vi "Serial_Write_Read_xbox_Polling.vi"() -> ()   [LabVIEW 2023]
uses:
  <vilib>/MakerHub/Xbox-One-Controller/Private/Type Defs/Indicators/Controller.ctl
  <vilib>/MakerHub/Xbox-One-Controller/Private/Type Defs/Indicators/A.ctl
  <vilib>/MakerHub/Xbox-One-Controller/Private/Type Defs/Indicators/B.ctl
  <vilib>/MakerHub/Xbox-One-Controller/Private/Type Defs/Indicators/X.ctl
  <vilib>/MakerHub/Xbox-One-Controller/Private/Type Defs/Indicators/Y.ctl
  <vilib>/MakerHub/Xbox-One-Controller/Private/Type Defs/Indicators/Left Bumper.ctl
  <vilib>/MakerHub/Xbox-One-Controller/Private/Type Defs/Indicators/Right Bumper.ctl
  <vilib>/MakerHub/Xbox-One-Controller/Private/Type Defs/Indicators/View.ctl
  <vilib>/MakerHub/Xbox-One-Controller/Private/Type Defs/Indicators/Menu.ctl
  <vilib>/MakerHub/Xbox-One-Controller/Private/Type Defs/Indicators/Thumbstick_Analog.ctl
  <vilib>/MakerHub/Xbox-One-Controller/Private/Type Defs/Indicators/Slider.ctl
  <vilib>/MakerHub/Xbox-One-Controller/Private/Type Defs/Indicators/DPad.ctl
  <vilib>/MakerHub/Xbox-One-Controller/Public/Open First Controller.vi
  <vilib>/Instr/_visa.llb/VISA Configure Serial Port (Instr).vi
  <vilib>/MakerHub/Xbox-One-Controller/LMH-Xbox-One-Controller.lvlib
panel:
  in  "Left Stick":u32(slide)=50 scale=0.0..100.0
  out "Loop Timer":i32
  out "Panel Outputs\nActive":bool
  in  "Right Bumper":T1 caption="Blank Button"
  in  "Left Bumper":T2 caption="Blank Button"
  in  "Menu Button":T3 caption="Blank Button"
  in  "View Button":T4 caption="Blank Button"
  in  "Y":T5 caption="Blank Button"
  in  "X":T6 caption="Blank Button"
  in  "B":T7 caption="Blank Button"
  in  "A":T8 caption="Blank Button"
  in  "Right Stick":u32(slide)=50 scale=0.1..100.0
  in  "Panel Buttons / Xbox Buttons":bool
  out "Controller":T9={"A Button"=FALSE, "B Button"=FALSE, "X Button"=FALSE, "Y Button"=FALSE, "Left Bumper"=FALSE, "Right Bumper"=FALSE, "View Button"=FALSE, "Menu Button"=FALSE, "Left Stick"={[], []}, "Right Stick"={[], []}, "Trigger"=0, "D-Pad"=5} {"Trigger" scale=32767.0..-32768.0}
  out "X Axis Right":u32
  out "X Axis Left":u32
  out "error out":errorcluster
  in  "error in (no error)":errorcluster
  in  "byte count\nRead":u32=40
  in  "Loop Timer":u32=100 min=10
  out "Concatenated \nNumber":string
  in  "VISA resource name":refnum<visa-resource-name>="COM3"
  out "byte count Sent":u32
  out "read buffer":string
  out "Controller Outputs\nActive":bool
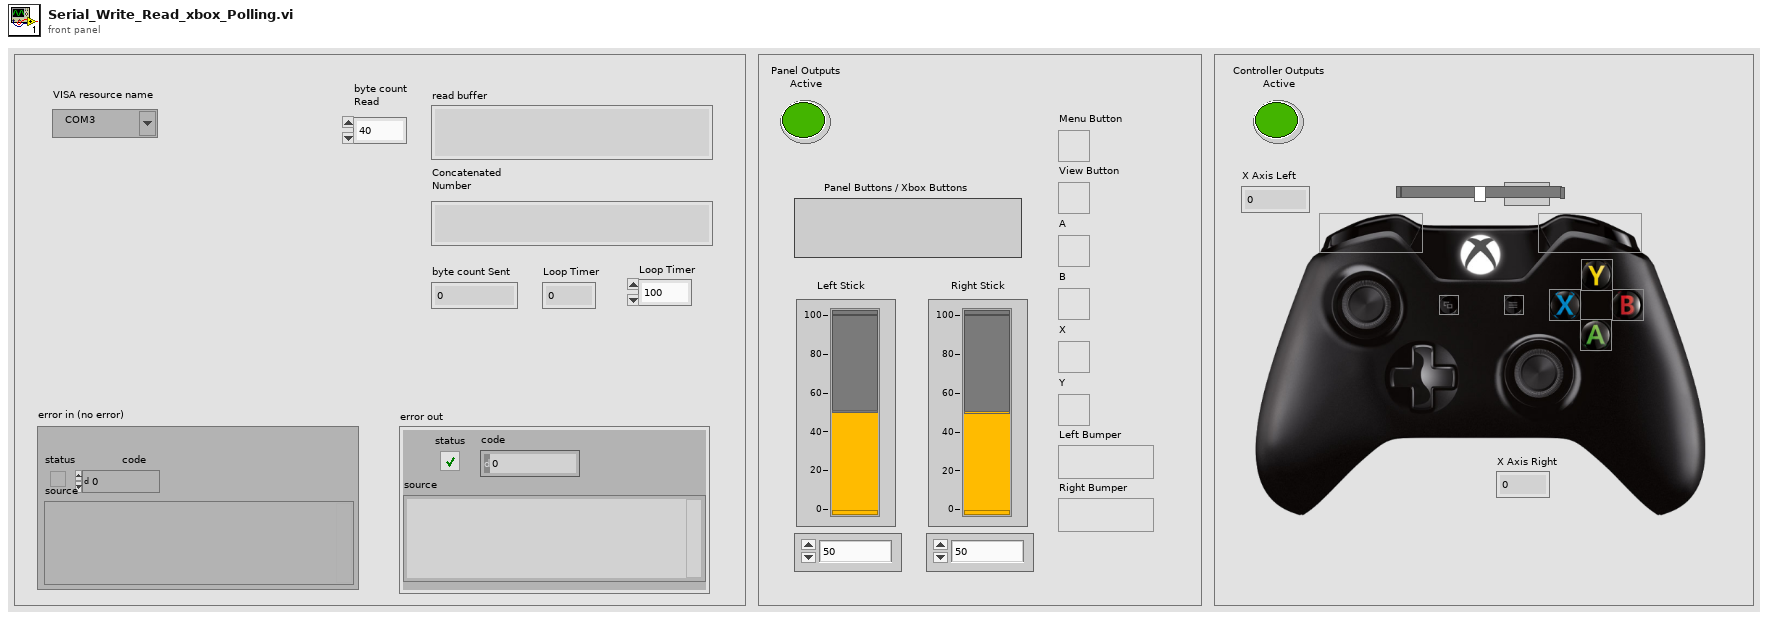
[diagram p1: front panel]
types:
  T1 = typedef "LMH-Xbox-One-Controller.lvlib/Right Bumper.ctl" = bool
  T2 = typedef "LMH-Xbox-One-Controller.lvlib/Left Bumper.ctl" = bool
  T3 = typedef "LMH-Xbox-One-Controller.lvlib/Menu.ctl" = bool
  T4 = typedef "LMH-Xbox-One-Controller.lvlib/View.ctl" = bool
  T5 = typedef "LMH-Xbox-One-Controller.lvlib/Y.ctl" = bool
  T6 = typedef "LMH-Xbox-One-Controller.lvlib/X.ctl" = bool
  T7 = typedef "LMH-Xbox-One-Controller.lvlib/B.ctl" = bool
  T8 = typedef "LMH-Xbox-One-Controller.lvlib/A.ctl" = bool
  T9 = typedef "LMH-Xbox-One-Controller.lvlib/Controller.ctl" = cluster{"A Button":T8, "B Button":T7, "X Button":T6, "Y Button":T5, "Left Bumper":T2, "Right Bumper":T1, "View Button":T4, "Menu Button":T3, "Left Stick":T10, "Right Stick":T10, "Trigger":T11, "D-Pad":T12}
  T10 = typedef "LMH-Xbox-One-Controller.lvlib/Thumbstick_Analog.ctl" = cluster{i32[], i32[]}
  T11 = typedef "LMH-Xbox-One-Controller.lvlib/Slider.ctl" = i32
  T12 = typedef "LMH-Xbox-One-Controller.lvlib/DPad.ctl" = u16
  T13 = typedef "LMH-Xbox-One-Controller.lvlib/Xbox One Controller Ref.ctl" = cluster{"Controller Ref":refnum<k1>, "Event Refnum":refnum<event-registration>, "Worker Ref":refnum<vi>}
  T14 = typedef "LMH-Xbox-One-Controller.lvlib/All Axis Data.ctl" = cluster{"Left Stick":cluster{"X Axis":i32, "Y Axis":i32}, "Right Stick":cluster{"X Axis":i32, "Y Axis":i32}, "Triggers":i32, "D-Pad":T15}
  T15 = typedef "LMH-Xbox-One-Controller.lvlib/DPad Enum.ctl" = enum16{"Idle", "Up", "Up / Right", "Right", "Down / Right", "Down", "Down / Left", "Left", "Up / Left"}
  T16 = typedef "LMH-Xbox-One-Controller.lvlib/All Buttons Visual.ctl" = cluster{"A":T8, "B":T7, "X":T6, "Y":T5, "Left Bumper":T2, "Right Bumper":T1, "View Button":T4, "Menu Button":T3, "Left Stick":T17, "Right Stick":T17}
  T17 = typedef "LMH-Xbox-One-Controller.lvlib/Thumbstick.ctl" = bool
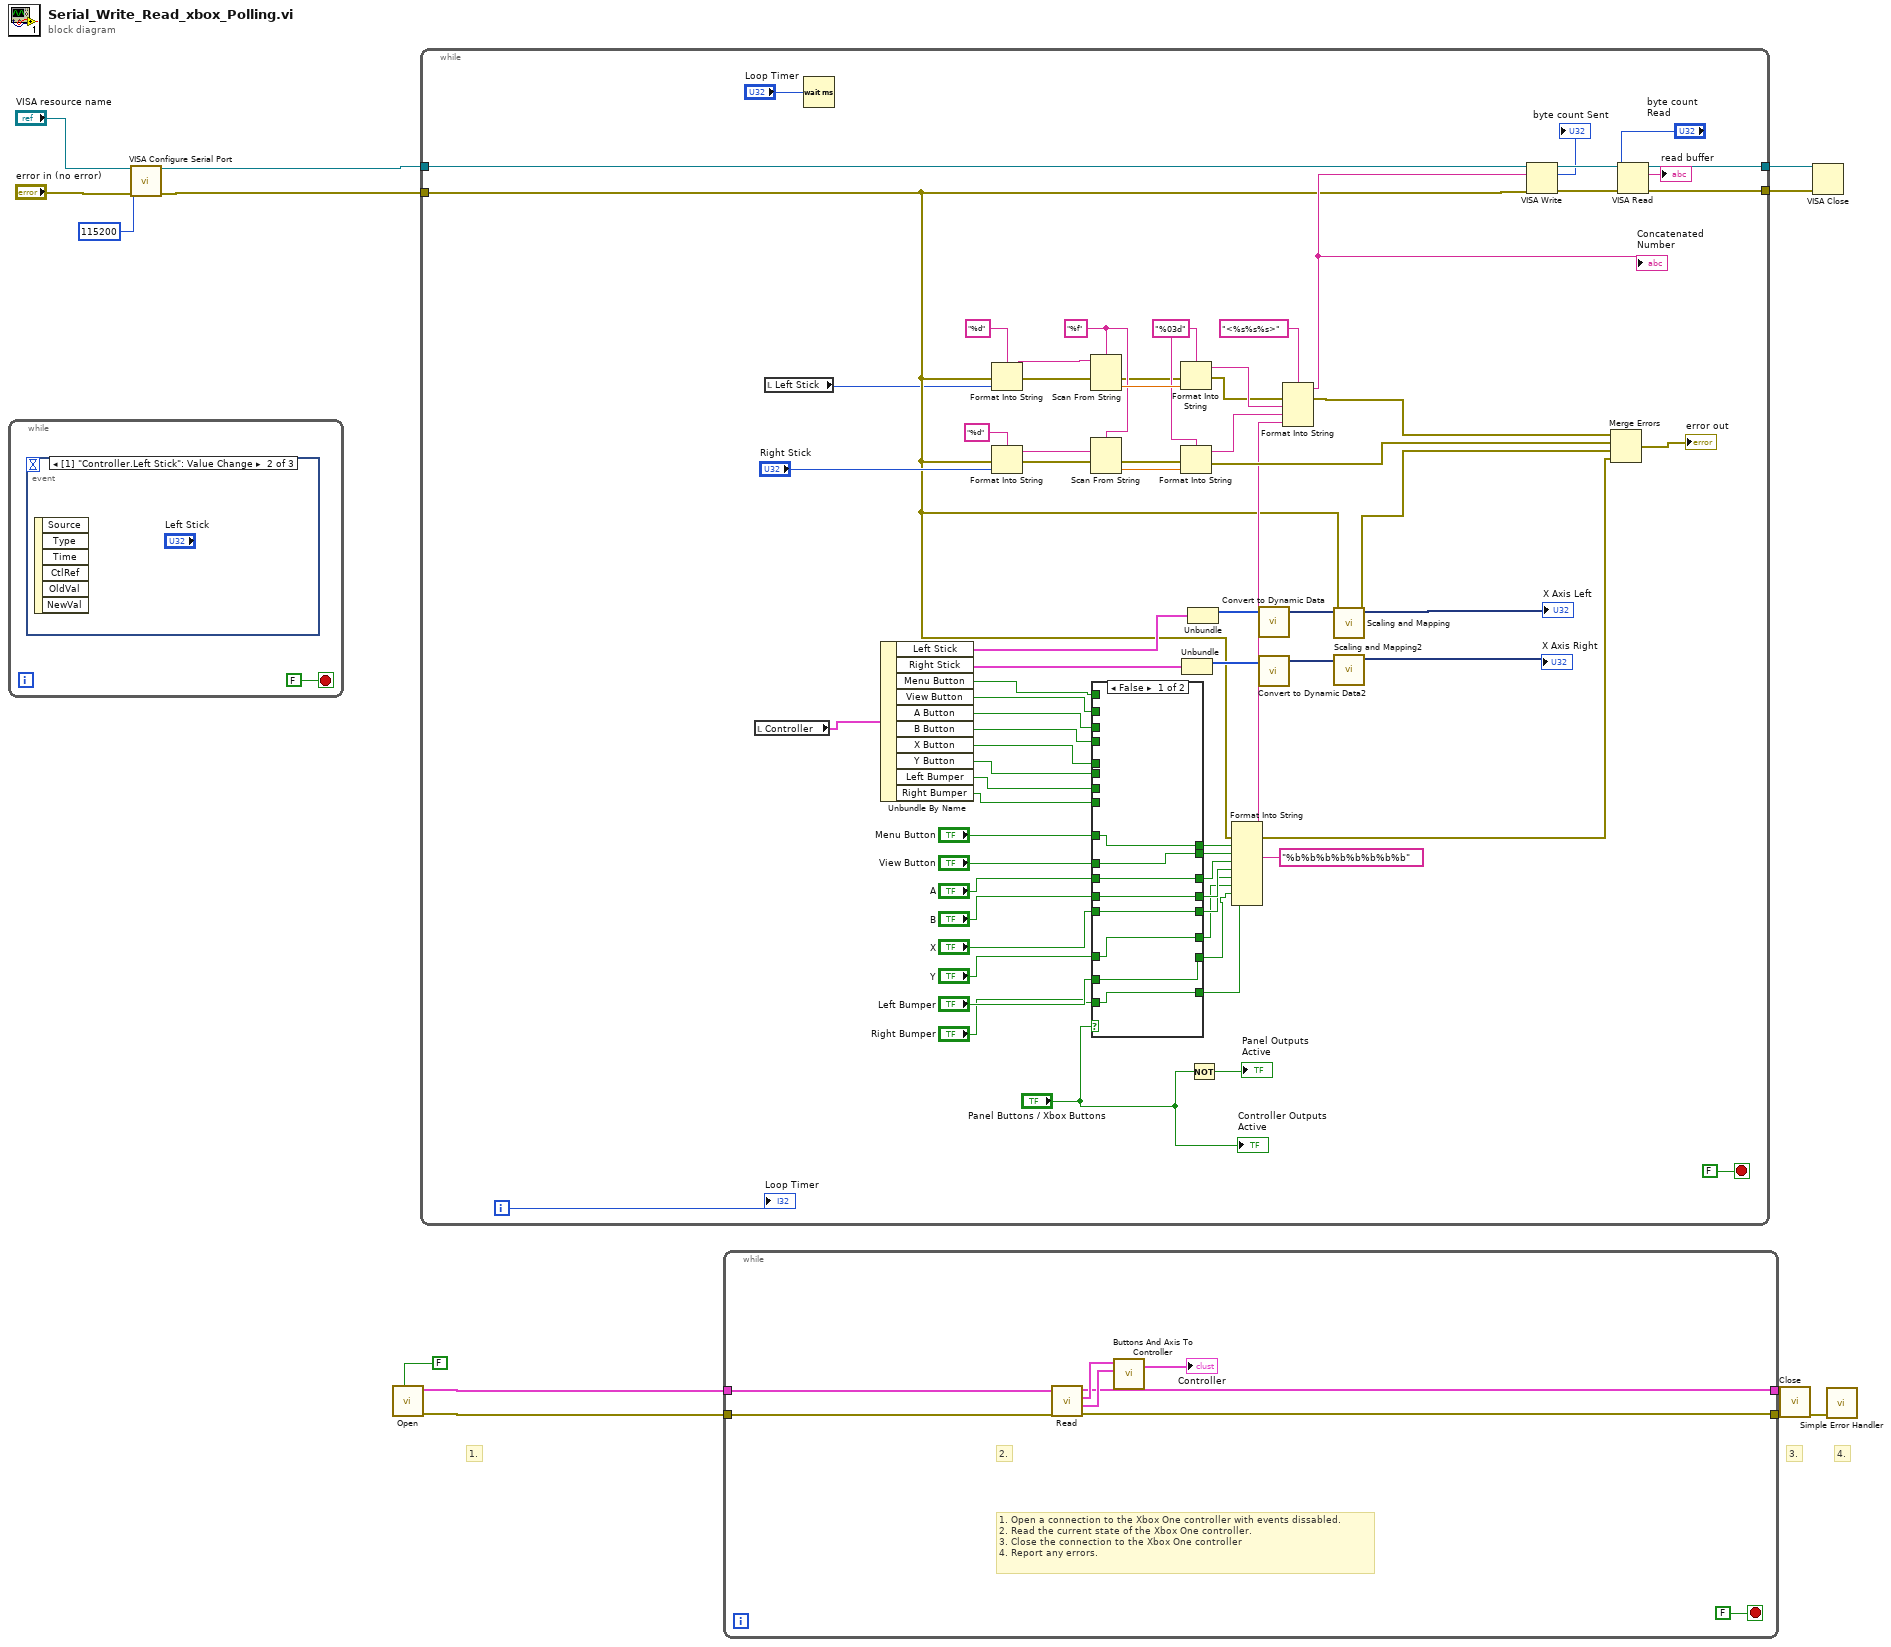
[diagram p0: block diagram]
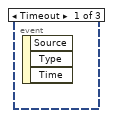
[diagram p2: hidden frame]
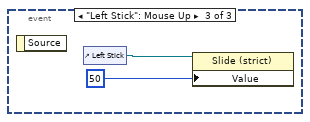
[diagram p3: hidden frame]
diagram:
  # "4."
  # "3."
  # "1."
  n1 = while {
    stop <- FALSE stop-if-true
    n2 = event shown="[1] \"Controller.Left Stick\": Value Change" {
      selector: _ -> [_ _ _]
      dyn-events: _ -> [_ _ _]
      timeout: _ -> [_ _ _]
      event Timeout {
        n3 = event-data() -> ()  [unwired: 1 in, 3 out]
      }
      event Value Change {
        n4 = event-data() -> ()  [unwired: 1 in, 6 out]
      }
      event "Left Stick": Mouse Up {
        n5 = event-data() -> ()  [unwired: 1 in, 1 out]
        n6 = control-ref of="Left Stick"() -> (w16:refnum<vi>)
        n7 = property class="Slide (strict)"(reference=w16, "Value"=u32 50) -> ()  [unwired: 1 in, 2 out]
      }
    }
  }
  n8 = call-poly "VISA Configure Serial Port"("VISA resource name"="VISA resource name", "baud rate (9600)"=u32 115200, "error in (no error)"="error in (no error)") -> ("VISA resource name out"=w11:refnum<visa-resource-name>, "error out"=w10:errorcluster)  [unwired: 11 in]
  n9 = call-poly <vilib>:"Open.vi"("Enable Events (T)"=FALSE) -> ("Error Out"=w4:errorcluster, "Xbox One Controller"=w3:T13)  [unwired: 8 in, 1 out]
  n10 = while {
    tunnel: [w88] -> w13
    tunnel: [w86] -> w12
    tunnel: w11 -> [w83]
    tunnel: w10 -> [w24]
    i -> [w22]
    stop <- FALSE stop-if-true
    w73 = "%f" ("format string")
    w75 = "%03d" ("format string")
    n11 = local read "Controller"() -> (w21:T9)
    n12 = local read "Left Stick"() -> (w17:u32)
    n13 = Wait (ms)(milliseconds to wait="Loop Timer") -> ()  [unwired: 1 out]
    n14 = Unbundle By Name(w21) -> ("Left Stick"=w60:T10, "Right Stick"=w59:T10, "Menu Button"=w33:T3, "View Button"=w32:T4, "A Button"=w31:T8, "B Button"=w30:T7, "X Button"=w29:T6, "Y Button"=w28:T5, "Left Bumper"=w27:T2, "Right Bumper"=w26:T1)
    n15 = Format Into String(format string="%d", error in=w24, w17) -> (resulting string=w79:string, error out=w68:errorcluster)  [unwired: 1 in]
    n16 = Format Into String(format string="%d", error in=w24, "Right Stick") -> (resulting string=w74:string, error out=w65:errorcluster)  [unwired: 1 in]
    n17 = Scan From String(format string=w73, input string=w79, error in=w68) -> (error out=w67:errorcluster, output 1=w80:dbl)  [unwired: 2 in, 2 out]
    n18 = Scan From String(format string=w73, input string=w74, error in=w65) -> (error out=w64:errorcluster, output 1=w70:dbl)  [unwired: 2 in, 2 out]
    n19 = case shown="False" "Panel Buttons / Xbox Buttons" {
      tunnel: "Menu Button" -> [w97 _]
      tunnel: [w97 w105] -> w48
      tunnel: "View Button" -> [w96 _]
      tunnel: [w96 w104] -> w46
      tunnel: "A" -> [w95 _]
      tunnel: [w95 w103] -> w44
      tunnel: "B" -> [w94 _]
      tunnel: "X" -> [w93 _]
      tunnel: "Y" -> [w92 _]
      tunnel: "Left Bumper" -> [w91 _]
      tunnel: "Right Bumper" -> [w90 _]
      tunnel: [w94 w102] -> w38
      tunnel: [w93 w101] -> w37
      tunnel: [w92 w100] -> w36
      tunnel: [w91 w99] -> w35
      tunnel: [w90 w98] -> w34
      tunnel: w33 -> [_ w105]
      tunnel: w32 -> [_ w104]
      tunnel: w31 -> [_ w103]
      tunnel: w30 -> [_ w102]
      tunnel: w29 -> [_ w101]
      tunnel: w28 -> [_ w100]
      tunnel: w27 -> [_ w99]
      tunnel: w26 -> [_ w98]
      frame False {
      }
      frame True {
      }
    }
    n20 = Format Into String(format string=w75, error in=w67, w80) -> (resulting string=w78:string, error out=w66:errorcluster)  [unwired: 1 in]
    n21 = Format Into String(format string=w75, error in=w64, w70) -> (resulting string=w76:string, error out=w62:errorcluster)  [unwired: 1 in]
    n22 = Unbundle(w59) -> (w54:i32[])  [unwired: 1 out]
    n23 = Unbundle(w60) -> (w58:i32[])  [unwired: 1 out]
    n24 = Not(x="Panel Buttons / Xbox Buttons") -> (.not. x?=→"Panel Outputs\nActive":bool)
    n25 = Format Into String(format string="%b%b%b%b%b%b%b%b", error in=w24, w48, w46, w44, w38, w37, w36, w35, w34) -> (resulting string=w51:string, error out=w23:errorcluster)  [unwired: 1 in]
    n26 = call "Convert to Dynamic Data"("Array"=w58) -> ("Dynamic Data Type"=w55:dynamicdata)  [unwired: 3 in]
    n27 = call "Convert to Dynamic Data2"("Array"=w54) -> ("Dynamic Data Type"=w53:dynamicdata)  [unwired: 3 in]
    n28 = Format Into String(format string="<%s%s%s>", error in=w66, w78, w76, w51) -> (resulting string=w69:string, error out=w63:errorcluster)  [unwired: 1 in]
    "Concatenated \nNumber" <- w69
    n29 = call "Scaling and Mapping"("error in (no error)"=w24, "Signals"=w55) -> ("error out"=w56:errorcluster, "Scaled Signals"=→"X Axis Left":dynamicdata)  [unwired: 8 in]
    n30 = call "Scaling and Mapping2"("Signals"=w53) -> ("Scaled Signals"=→"X Axis Right":dynamicdata)  [unwired: 9 in, 1 out]
    n31 = VISA Write(VISA resource name=w83, write buffer=w69, error in (no error)=w24) -> (VISA resource name out=w89:refnum<visa-resource-name>, return count=→"byte count Sent":u32, error out=w85:errorcluster)
    n32 = Merge Errors(w63, w62, w56, w23) -> (→"error out":errorcluster)
    n33 = VISA Read(VISA resource name=w89, byte count="byte count\nRead", error in (no error)=w85) -> (VISA resource name out=w88:refnum<visa-resource-name>, read buffer=→"read buffer":string, error out=w86:errorcluster)  [unwired: 1 out]
    "Controller Outputs\nActive" <- "Panel Buttons / Xbox Buttons"
    "Loop Timer" <- w22
  }
  n34 = while {
    tunnel: w4 -> [w113]
    tunnel: w3 -> [w108]
    tunnel: [w110] -> w7
    tunnel: [w109] -> w6
    stop <- FALSE stop-if-true
    # "1. Open a connection to the Xbox One controller with events dissabled.\n2. Read the current state of the Xbox One controller.\n3. Close the connection to the Xbox One controller\n4. Report any errors."
    # "2."
    n35 = call <vilib>:"Read.vi"("Error In"=w113, "Xbox One Controller Ref"=w108) -> ("Error Out"=w109:errorcluster, "All Axis"=w111:T14, "Buttons"=w112:T16, "Xbox One Controller Ref"=w110:T13)  [unwired: 6 in]
    n36 = call <vilib>:"Buttons And Axis To Controller.vi"("All Axis"=w111, "Buttons"=w112) -> ("Controller"=→"Controller":T9)  [unwired: 5 in]
  }
  n37 = call <vilib>:"Close.vi"("Error In"=w6, "Xbox One Controller Ref"=w7) -> ("Error Out"=w5:errorcluster)  [unwired: 9 in]
  n38 = VISA Close(VISA resource name=w13, error in (no error)=w12) -> ()  [unwired: 1 out]
  n39 = call <vilib>:"Simple Error Handler.vi"("error in (no error)"=w5) -> ()  [unwired: 4 in, 5 out]
